vi "Check valid sensor.vi"(8 "Geometry in":string, 9 "Resolution in":string, 10 "Thickness in":string, 11 "Sensor ID":string) -> (0 "Geometry out":string, 1 "Resolution out":string, 2 "Thickness out":string, 3 "Sensor ID out":string, 4 "Sensor ID okay":bool)   [LabVIEW 2021, in "Database Entry.lvclass"]
uses:
  Database Entry.lvclass
  <vilib>/Utility/file.llb/Read Delimited Spreadsheet (string).vi
  <vilib>/JDP Science/JDP Science Common Utilities/JDP Utility.lvlib
panel:
  out "sensor_geometry":string[][](array[string])
  out "Returned":string[](array[string])
  out "first digits":string[](array[string])
  out "sensor_thickness_resolution_type":string[][](array[string])
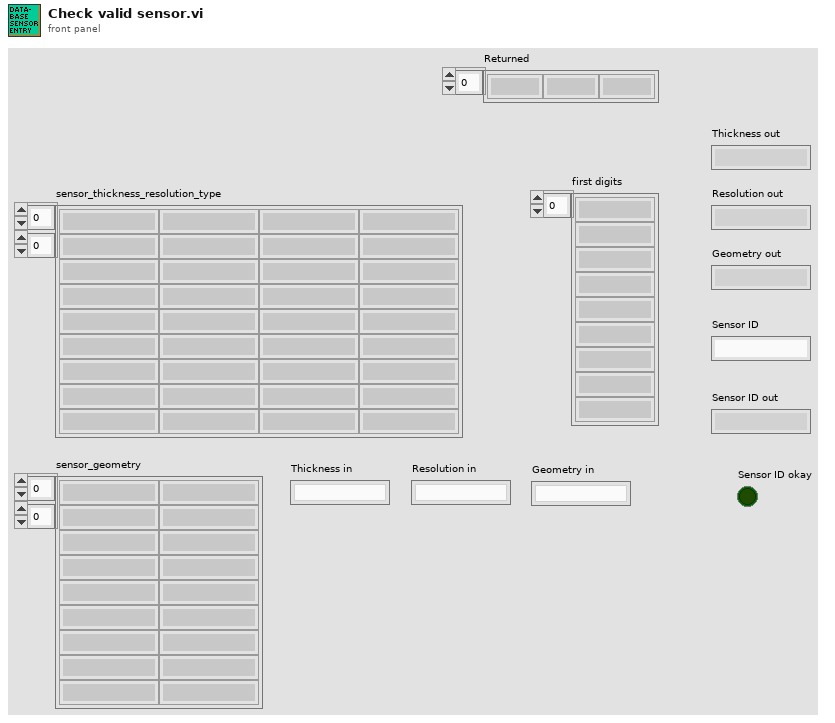
[diagram p1: front panel]
types:
  T1 = typedef "File Paths.ctl" = cluster{"Glue Pattern Folder":path, "Carrier Tray Folder":path, "Pick Up Tool Fixture Folder":path, "Components Folder":path, "Bellows Tool Offset.txt":path, "Pick Up Tool Offset.txt":path, "Dispense Tip Offset.txt":path, "Log Files":path, "Gantry Assembly Map.txt":path, "Syringe and offset map.txt":path, "Controllers Folder":path, "Local dbase config":path}
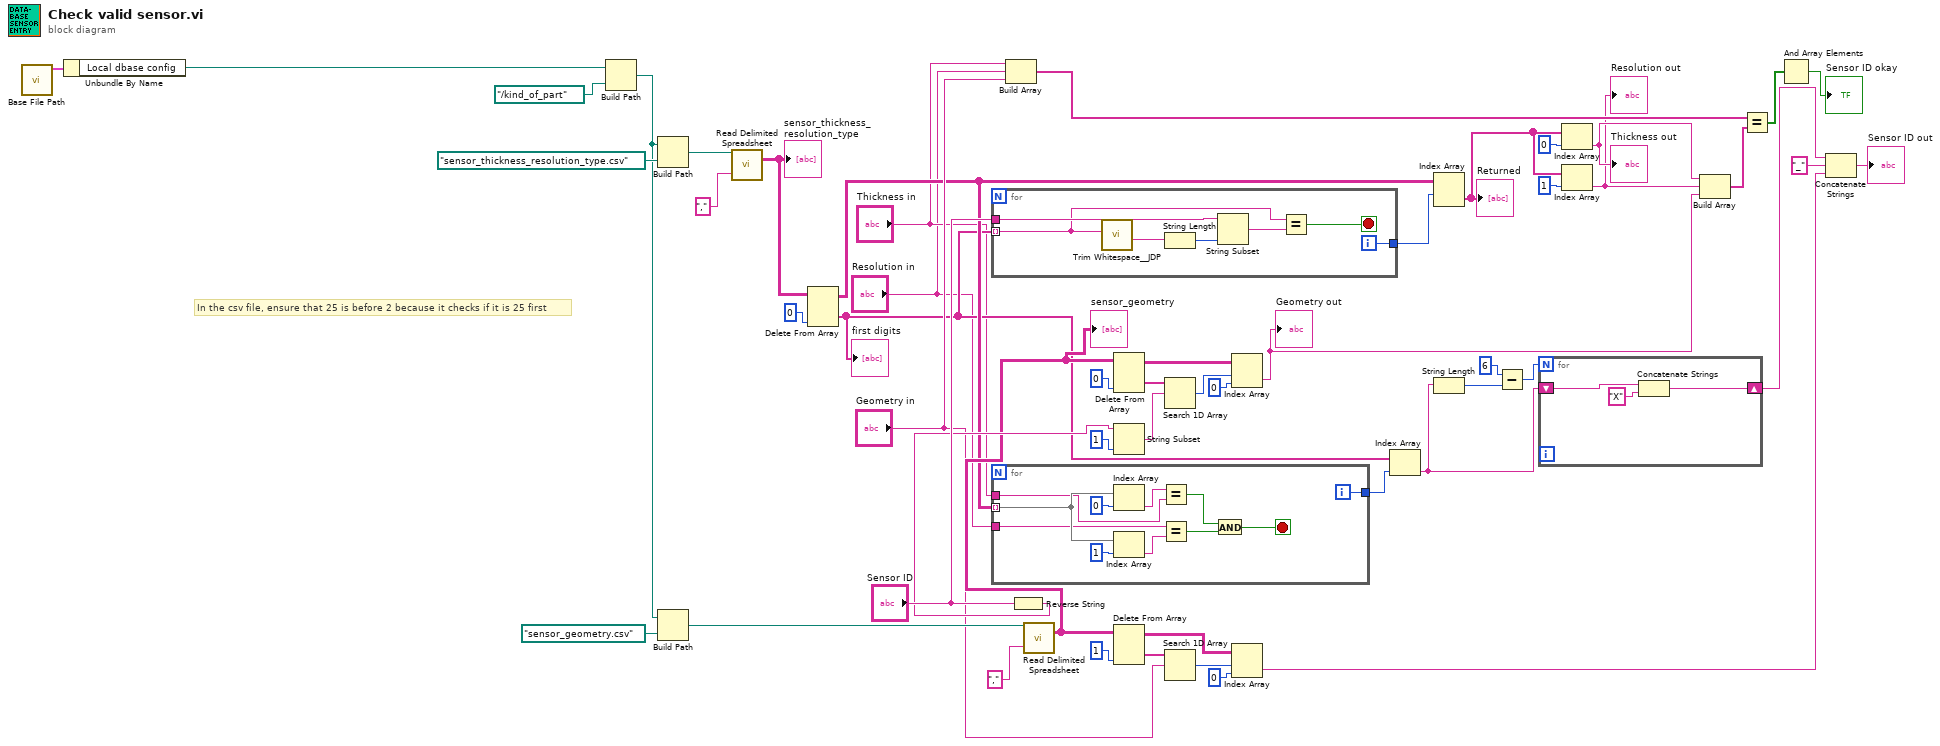
[diagram p0: block diagram]
diagram:
  # "In the csv file, ensure that 25 is before 2 because it checks if it is 25 first"
  n1 = call "Base File Path.vi"() -> ("Paths Out"=w50:T1)  [unwired: 11 in]
  n2 = Unbundle By Name(w50) -> ("Local dbase config"=w49:path)
  n3 = Build Path(base path=w49, name or relative path=path "../kind_of_part") -> (appended path=w44:path)
  n4 = Build Path(base path=w44, name or relative path=path "sensor_thickness_resolution_type.csv") -> (appended path=w51:path)
  n5 = Build Path(base path=w44, name or relative path=path "sensor_geometry.csv") -> (appended path=w43:path)
  n6 = call-poly <vilib>:"Read Delimited Spreadsheet.vi"("file path (dialog if empty)"=w51, "delimiter (\\t)"="," ("delimiter (\\t)")) -> ("all rows"=w46:string[][])  [unwired: 8 in, 5 out]
  "sensor_thickness_resolution_type" <- w46
  n7 = Delete From Array(array=w46, index (col)=0 ("disabled index (col)")) -> (deleted portion=w9:string[], array with subset deleted=w10:string[][])  [unwired: 2 in]
  "first digits" <- w9
  n8 = for {
    tunnel: w9 -> [w54] mode=indexing
    tunnel: "Sensor ID" -> [w57]
    tunnel: [w53] -> w38
    i -> [w53]
    stop <- w56 stop-if-true
    n9 = call <vilib>:"Trim Whitespace__JDP.vi"("String in"=w54) -> ("String out"=w59:string)  [unwired: 6 in]
    n10 = String Length(string=w59) -> (length=w58:i32)
    n11 = String Subset(string=w57, length (rest)=w58) -> (substring=w55:string)  [unwired: 1 in]
    n12 = Equal?(x=w54, y=w55) -> (x = y?=w56:bool)
  }
  n13 = for {
    tunnel: w10 -> [w70] mode=indexing
    tunnel: [w67] -> w8
    tunnel: "Thickness in" -> [w61]
    tunnel: "Resolution in" -> [w60]
    i -> [w67]
    stop <- w62 stop-if-true
    n14 = Index Array(array=w70, index=0) -> (element=w66:string)
    n15 = Index Array(array=w70, index=1) -> (element=w65:string)
    n16 = Equal?(x=w66, y=w61) -> (x = y?=w64:bool)
    n17 = Equal?(x=w60, y=w65) -> (x = y?=w63:bool)
    n18 = And(x=w64, y=w63) -> (x .and. y?=w62:bool)
  }
  n19 = Build Array("Thickness in", "Resolution in", "Geometry in") -> (w27:string[])
  n20 = Reverse String(1:"Sensor ID") -> (0:w33:string)
  n21 = call-poly <vilib>:"Read Delimited Spreadsheet.vi"("file path (dialog if empty)"=w43, "delimiter (\\t)"="," ("delimiter (\\t)")) -> ("all rows"=w19:string[][])  [unwired: 8 in, 5 out]
  "sensor_geometry" <- w19
  n22 = Delete From Array(array=w19, index (col)=0 ("disabled index (col)")) -> (deleted portion=w31:string[], array with subset deleted=w30:string[][])  [unwired: 2 in]
  n23 = String Subset(string=w33, length (rest)=1 ("length (rest)")) -> (substring=w32:string)  [unwired: 1 in]
  n24 = Delete From Array(array=w19, index (col)=1) -> (deleted portion=w18:string[], array with subset deleted=w16:string[][])  [unwired: 2 in]
  n25 = Search 1D Array(1D array=w31, element=w32) -> (index of element=w29:i32)  [unwired: 1 in]
  n26 = Search 1D Array(1D array=w18, element="Geometry in") -> (index of element=w14:i32)  [unwired: 1 in]
  n27 = Index Array(array=w30, index (row)=w29, index (col)=0 ("disabled index (row)")) -> (element=w24:string)
  "Geometry out" <- w24
  n28 = Index Array(array=w16, index (row)=w14, index (col)=0 ("disabled index (col)")) -> (element=w12:string)
  n29 = Index Array(array=w9, index=w8) -> (element=w2:string)
  n30 = Index Array(array=w10, index (row)=w38) -> (element=w37:string[])  [unwired: 1 in]
  "Returned" <- w37
  n31 = String Length(string=w2) -> (length=w5:i32)
  n32 = Subtract(x=6, y=w5) -> (x-y=w3:i32)
  n33 = for {
    N: w3 -> [_]
    shift-right: [w71] -> w1
    shift-left: w2 -> [w73]
    n34 = Concatenate Strings(w73, "X" ("string")) -> (w71:string)
  }
  n35 = Index Array(array=w37, index=0) -> (element=w26:string)
  "Thickness out" <- w26
  n36 = Index Array(array=w37, index=1) -> (element=w25:string)
  "Resolution out" <- w25
  n37 = Build Array(w26, w25, w24) -> (w23:string[])
  n38 = Equal?(x=w27, y=w23) -> (x = y?=w22:bool[])
  n39 = And Array Elements(Boolean array=w22) -> (logical AND=→"Sensor ID okay":bool)
  n40 = Concatenate Strings(w1, "_" ("string"), w12) -> (→"Sensor ID out":string)
